vi "Write GObject selectors.vi"(8 "Error in":errorcluster, 10 "Selectors":string[](array[string]), 11 "GObject in":refnum<vi>) -> (0 "Error out":errorcluster)   [LabVIEW 2019, in "LSS.lvlib"]
doc: "Write the selectors into the \"Selectors\" tag of the front panel object. These selectors are used to determine which properties apply to which controls.\n\n<b>Inputs:</b>\n<b>GObject in</b> - Object that will have it's \"Selectors\" tag modified.\n<b>Selectors</b> - List of selectors that apply to specific object referenced by GObject in.\n<b>Error In</b> - Standard Error In terminal.\n\n<b>Outputs:</b>\n<b>Error Out</b> - Standard Error Out terminal."
uses:
  LSS.lvlib
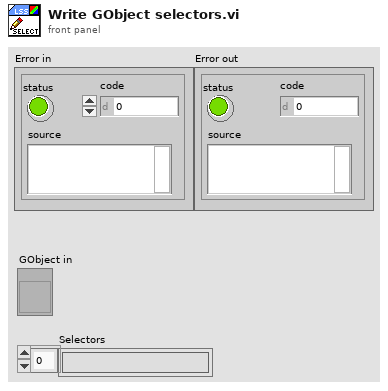
[diagram p1: front panel]
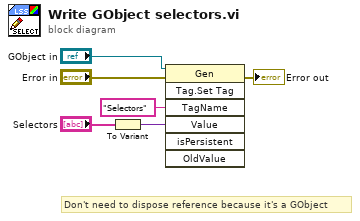
[diagram p0: block diagram]
diagram:
  # "Don't need to dispose reference because it's a GObject"
  n1 = To Variant(anything="Selectors") -> (Variant=w6:variant)
  n2 = invoke class="Gen" method="Tag.Set Tag"(reference="GObject in", error in="Error in", "TagName"="Selectors" ("Tag Name"), "Value"=w6) -> (error out=→"Error out":errorcluster)  [unwired: 3 in, 6 out]
